vi "Commercial Report (SubVI).vi"(4 "shotsArr":T3 {"Frag Rod" format="%.1f"; "UncorrectedAvgVel_PB" format="%.1f"; "UncorrectedRed_PB" format="%.1f"; "strikeVel_PB" format="%.1f"; "velLoss_PB" format="%.1f"; "avgVel_PB" format="%.1f"; "Redundant_Velocity" format="%.1f"; "Energy Loss (J)" format="%.3e"; "Projectile Mass" min=0 step=1 format="%.4f"; "Corrected residual" format="%.2f"; "Uncorrected Residual" format="%.1f"; "Corrected Impact" format="%.2f"; "Uncorrected Impact" format="%.1f"; "Shot Angle" max=90 step=1; "SHOT STATUS" items=["Partial", "Complete"]; "IMPACT VELOCITY" min=0 max=10000 step=0.1 format="%.1f"; "Barrel Temperature" format="%.1f"; "Powder Loading" format="%.4f"; "RESIDUAL  VELOCITY" min=0 max=10000 step=0.1 format="%.1f"}, 5 "V50 Data":T2, 6 "NIJ Data":T1, 7 "Common Data":T5, 8 "errIN":errorcluster, 9 "language":enum16{"Spanish", "Portuguese", "English"}(ring), 10 "reportType":enum32{"V50", "NIJ"}(radio), 11 "SampleID":string) -> (0 "errOUT":errorcluster, 3 "rptStat":string)   [LabVIEW 2015]
uses:
  shotsArr.ctl
  Shot Record.ctl
  <vilib>/Utility/NIReport.llb/Append Report Text (str wrap).vi
  <vilib>/Utility/NIReport.llb/NI_report.lvclass
panel:
  # "BIMS Collector label"
  # "name (excel)"
  # "BIMS Collector label"
  # "name (excel)"
  # "Corrected"
  # "BIMS Collector label"
  # "name (excel)"
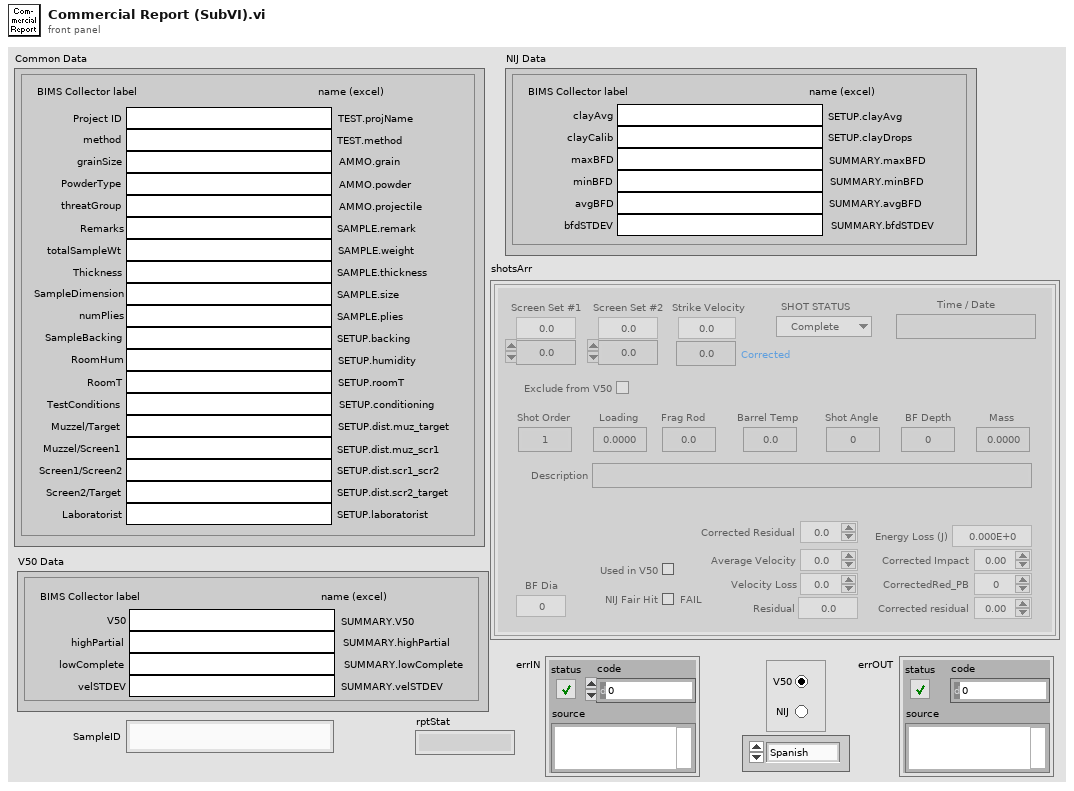
[diagram p1: front panel]
types:
  T1 = cluster{"SETUP.clayAvg":string, "SETUP.clayDrops":string, "SUMMARY.maxBFD":string, "SUMMARY.minBFD":string, "SUMMARY.avgBFD":string, "SUMMARY.bfdSTDEV":string}
  T2 = cluster{"SUMMARY.V50":string, "SUMMARY.highPartial":string, "SUMMARY.lowComplete":string, "SUMMARY.velSTDEV":string}
  T3 = typedef "shotsArr.ctl" = T4[]
  T4 = typedef "Shot Record.ctl" = cluster{"Uncorrected Impact":sgl, "Uncorrected Residual":sgl, "avgVel_PB":sgl, "IMPACT VELOCITY":sgl, "RESIDUAL  VELOCITY ":sgl, "Shot Description":string, "Powder Loading ":sgl, "Barrel Temperature":sgl, "TIME / DATE":string, "shot order":i32, "SHOT STATUS":u16, "Shot Angle":u16, "Corrected Impact":sgl, "Corrected residual":sgl, "Projectile Mass":sgl, "usedv50":bool, "Energy Loss (J)":sgl, "BackFace\nDepth":sgl, "BackFace\nDiameter":sgl, "Redundant_Velocity":sgl, "velLoss_PB":sgl, "strikeVel_PB":sgl, "UncorrectedRed_PB":sgl, "CorrectedRed_PB":sgl, "UncorrectedAvgVel_PB":sgl, "V50userExcl":bool, "Frag Rod":sgl, "fairHit":bool}
  T5 = cluster{"TEST.projName":string, "SAMPLE.remark":string, "TEST.method":string, "SAMPLE.thickness":string, "SAMPLE.size":string, "SAMPLE.plies":string, "AMMO.powder":string, "SETUP.backing":string, "SAMPLE.weight":string, "SETUP.humidity":string, "SETUP.roomT":string, "AMMO.grain":string, "AMMO.projectile":string, "SETUP.conditioning":string, "SETUP.dist.muz_target":string, "SETUP.dist.muz_scr1":string, "SETUP.dist.scr1_scr2":string, "SETUP.dist.scr2_target":string, "SETUP.laboratorist":string}
  T6 = cluster{"position (excel)":cluster{"row":i32, "column":i32}, "name (excel)":string, "bookmark (word)":string}
  T7 = enum16{"maximized", "minimized", "normal", "no change"}
  T8 = enum16{"Standard Report", "HTML", "Word", "Excel"}
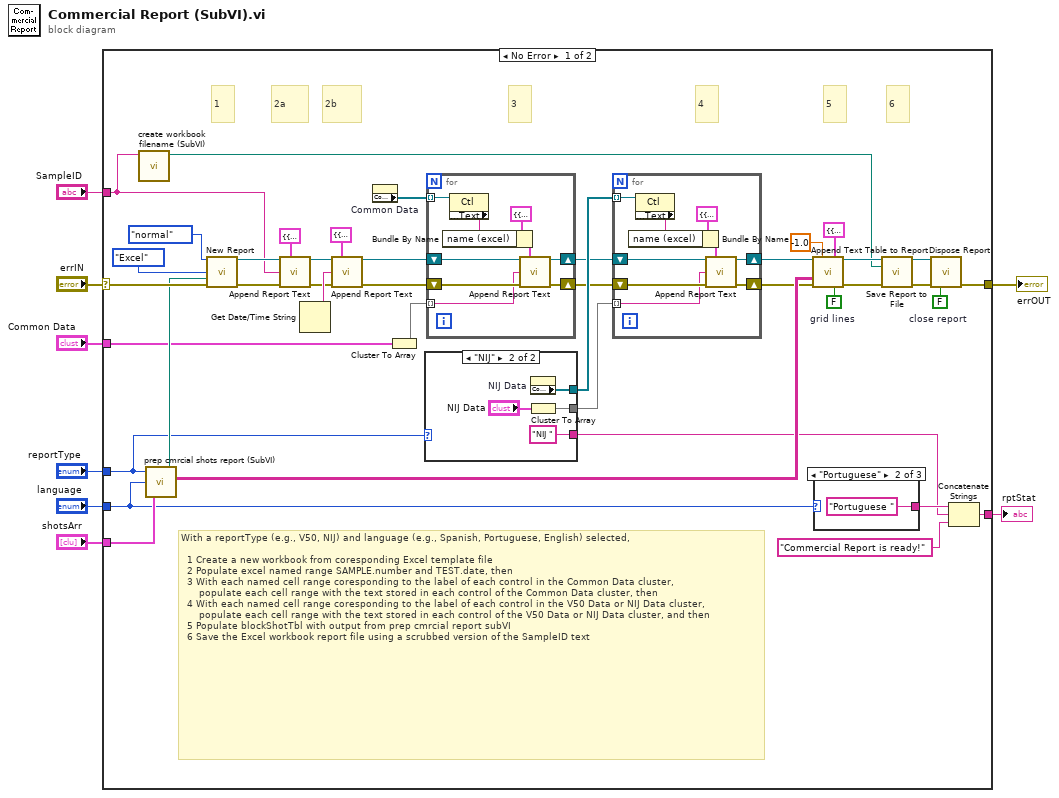
[diagram p0: block diagram]
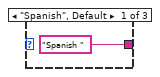
[diagram p2: hidden frame]
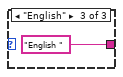
[diagram p3: hidden frame]
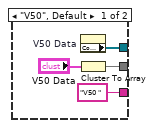
[diagram p4: hidden frame]
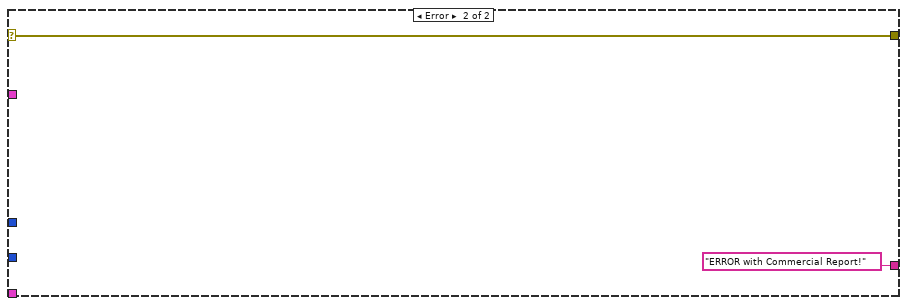
[diagram p5: hidden frame]
diagram:
  n1 = case shown="No Error" "errIN" {
    selector: "errIN" -> [w37 w80]
    tunnel: [w47 w80] -> w8
    tunnel: "language" -> [w13 _]
    tunnel: "reportType" -> [w20 _]
    tunnel: "SampleID" -> [w24 _]
    tunnel: "shotsArr" -> [w23 _]
    tunnel: "Common Data" -> [w22 _]
    tunnel: [w10 "ERROR with Commercial Report!"] -> w1
    frame No Error {
      w32 = FALSE  # grid lines
      w42 = FALSE  # close report
      # "With a reportType (e.g., V50, NIJ) and language (e.g., Spanish, Portuguese, English) selected,\n\n  1 Create a new workbook from coresponding Excel template file\n  2 Populate excel named range SAMPLE.number and TEST.date, then\n  3 With each named cell range coresponding to the label of each control in the Common Data cluster, \n      populate each cell range with the text stored in each control of the Common Data cluster, then\n  4 With each named cell range coresponding to the label of each control in the V50 Data or NIJ Data cluster, \n      populate each cell range with the text stored in each control of the V50 Data or NIJ Data cluster, and then\n  5 Populate blockShotTbl with output from prep cmrcial report subVI\n  6 Save the Excel workbook report file using a scrubbed version of the SampleID text"
      # "4"
      # "5"
      # "2a"
      # "2b"
      # "3"
      # "1"
      # "6"
      n2 = call "create workbook filename (SubVI).vi"("SampleID"=w24) -> ("Excel report workbook file name"=w21:path)  [unwired: 10 in]
      n3 = call "prep cmrcial shots report (SubVI).vi"("reportType"=w20, "language"=w13, "shotsArr"=w23) -> ("Custom Template"=w25:path, "shotArrayOUT"=w36:string[][])  [unwired: 2 in]
      n4 = call <vilib>:"New Report.vi"("window state (normal)"=T7."normal", "report type"=T8."Excel", "template (empty)"=w25, "error in (no error)"=w37) -> ("report out"=w29:refnum<class "NI_report.lvclass">, "error out"=w28:errorcluster)  [unwired: 10 in]
      n5 = call-poly <vilib>:"Append Report Text.vi"("report in"=w29, "MS Office parameters"=T6 {"position (excel)"={"row"=0, "column"=0}, "name (excel)"="SAMPLE.number", "bookmark (word)"=""}, "text"=w24, "error in (no error)"=w28) -> ("report out"=w26:refnum<class "NI_report.lvclass">, "error out"=w27:errorcluster)  [unwired: 8 in, 2 out]
      n6 = Get Date/Time String() -> (date string=w43:string)  [unwired: 3 in, 1 out]
      n7 = call-poly <vilib>:"Append Report Text.vi"("report in"=w26, "MS Office parameters"=T6 {"position (excel)"={"row"=0, "column"=0}, "name (excel)"="TEST.date", "bookmark (word)"=""}, "text"=w43, "error in (no error)"=w27) -> ("report out"=w41:refnum<class "NI_report.lvclass">, "error out"=w40:errorcluster)  [unwired: 8 in, 2 out]
      n8 = property on="Common Data" class="Clust (strict)"() -> ("Controls[]"=w38:refnum<vi>[])  [unwired: 2 in, 2 out]
      n9 = Cluster To Array(cluster=w22) -> (array=w39:string[])
      n10 = case shown="\"NIJ\"" w20 {
        tunnel: [w64 w68] -> w19
        tunnel: [w63 w67] -> w18
        tunnel: ["V50 " "NIJ "] -> w11
        frame "V50", Default {
          n11 = Cluster To Array(cluster="V50 Data") -> (array=w64:string[])
          n12 = property on="V50 Data" class="Clust (strict)"() -> ("Controls[]"=w63:refnum<vi>[])  [unwired: 2 in, 2 out]
        }
        frame "NIJ" {
          n13 = Cluster To Array(cluster="NIJ Data") -> (array=w68:string[])
          n14 = property on="NIJ Data" class="Clust (strict)"() -> ("Controls[]"=w67:refnum<vi>[])  [unwired: 2 in, 2 out]
        }
      }
      n15 = for {
        tunnel: w38 -> [w78] mode=indexing
        shift-right: [w74] -> w17
        shift-left: w41 -> [w73]
        shift-right: [w72] -> w16
        shift-left: w40 -> [w71]
        tunnel: w39 -> [w70] mode=indexing
        n16 = property class="Ctl"(reference=w78) -> ("Label.Text"=w76:string)  [unwired: 1 in, 2 out]
        n17 = Bundle By Name(cluster=T6 {"position (excel)"={"row"=0, "column"=0}, "name (excel)"="aCellRange", "bookmark (word)"=""} ("MS Office parameters"), "name (excel)"=w76) -> (w75:T6)
        n18 = call-poly <vilib>:"Append Report Text.vi"("report in"=w73, "MS Office parameters"=w75, "text"=w70, "error in (no error)"=w71) -> ("report out"=w74:refnum<class "NI_report.lvclass">, "error out"=w72:errorcluster)  [unwired: 8 in, 2 out]
      }
      n19 = for {
        tunnel: w18 -> [w61] mode=indexing
        shift-right: [w57] -> w14
        shift-left: w17 -> [w56]
        shift-right: [w55] -> w15
        shift-left: w16 -> [w54]
        tunnel: w19 -> [w53] mode=indexing
        n20 = property class="Ctl"(reference=w61) -> ("Label.Text"=w59:string)  [unwired: 1 in, 2 out]
        n21 = Bundle By Name(cluster=T6 {"position (excel)"={"row"=0, "column"=0}, "name (excel)"="aCellRange", "bookmark (word)"=""} ("MS Office parameters"), "name (excel)"=w59) -> (w58:T6)
        n22 = call-poly <vilib>:"Append Report Text.vi"("report in"=w56, "MS Office parameters"=w58, "text"=w53, "error in (no error)"=w54) -> ("report out"=w57:refnum<class "NI_report.lvclass">, "error out"=w55:errorcluster)  [unwired: 8 in, 2 out]
      }
      n23 = call-dynamic "Append Text Table to Report.vi"("report in"=w14, "column width (1)"=-1.0, "MS Office parameters"=T6 {"position (excel)"={"row"=0, "column"=0}, "name (excel)"="blockShotTbl", "bookmark (word)"=""}, "text data"=w36, "error in (no error)"=w15, "show grid lines (YES)"=w32) -> ("report out"=w34:refnum<class "NI_report.lvclass">, "error out"=w33:errorcluster)  [unwired: 6 in, 2 out]
      n24 = case shown="\"Portuguese\"" w13 {
        tunnel: ["Spanish " "Portuguese " "English "] -> w12
        frame "Spanish", Default {
        }
        frame "Portuguese" {
        }
        frame "English" {
        }
      }
      n25 = call-dynamic "Save Report to File.vi"("report in"=w34, "report file path"=w21, "error in (no error)"=w33) -> ("report out"=w46:refnum<class "NI_report.lvclass">, "error out"=w45:errorcluster)  [unwired: 11 in]
      n26 = call-dynamic "Dispose Report.vi"("report in"=w46, "error in (no error)"=w45, "close report? (T)"=w42) -> ("error out"=w47:errorcluster)  [unwired: 12 in]
      n27 = Concatenate Strings(w12, w11, "Commercial Report is ready!" ("message")) -> (w10:string)
    }
    frame Error {
    }
  }
  "errOUT" <- w8
  "rptStat" <- w1
